vi "Send Message.vi"(8 "error in (no error)":errorcluster, 10 "Message":T1, 11 "UDP Ref":refnum<k16>) -> (0 "error out":errorcluster, 3 "connection ID out":refnum<k16>)   [LabVIEW 2019]
uses:
  Message Globals.vi
  Typedefs/Sensor Types.ctl
  Typedefs/Message Types.ctl
  Typedefs/Message.ctl
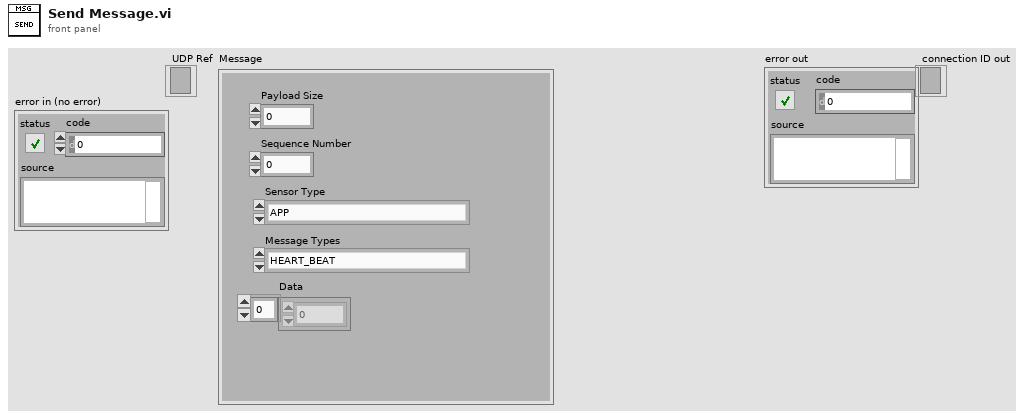
[diagram p1: front panel]
types:
  T1 = typedef "Message.ctl" = cluster{"Payload Size":u8, "Sequence Number":u8, "Sensor Type":T2, "Message Types":T3, "Data":u8[]}
  T2 = typedef "Sensor Types.ctl" = enum16{"APP", "TURBIDITY", "PH"}
  T3 = typedef "Message Types.ctl" = enum16{"HEART_BEAT", "CONNECT", "GET_CURRENT_MEASUREMENTS", "GET_LOG_FILE", "SEND_LOG_FILE_SIZE", "SEND_LOG_FILE_CHUNK", "GET_LOGGING_PERIOD", "SET_LOGGING_PERIOD", "SEND_SD_CARD_INFO", "GET_LOGS_LIST", "SEND_LOG_FILE_NAME", "SEND_LOGGING_PERIOD", "GET_RTC_TIME", "SET_RTC_TIME", "SEND_RTC_TIME", "SEND_CURRENT_MEASUREMENTS", "DELETE_LOG_FILE", "GET_SD_CARD_INFO", "GET_BATTERY_INFO", "SEND_BATTERY_INFO", "GET_LOG_FILE_SIZE", "ERROR_MSG"}
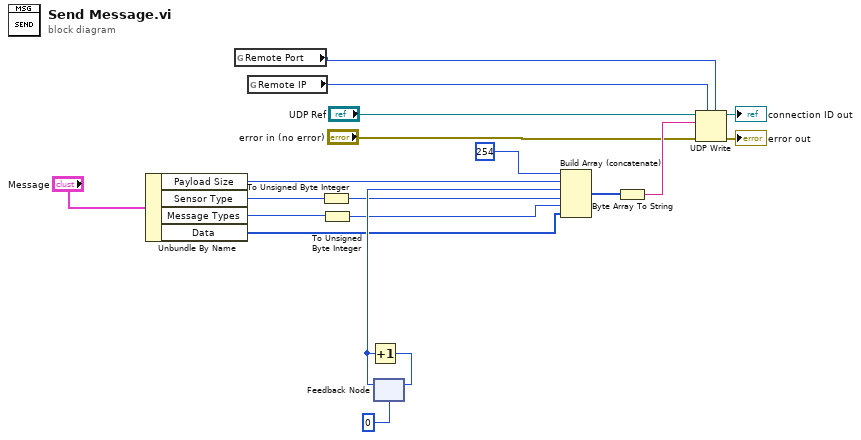
[diagram p0: block diagram]
diagram:
  n1 = Unbundle By Name("Message") -> ("Payload Size"=w9:u8, "Sensor Type"=w5:T2, "Message Types"=w3:T3, "Data"=w1:u8[])
  n2 = global read "Message Globals.vi" "Remote Port"() -> (w13:u16)
  n3 = global read "Message Globals.vi" "Remote IP"() -> (w14:u32)
  n4 = To Unsigned Byte Integer(number=w5) -> (unsigned 8bit integer=w4:u8)
  n5 = To Unsigned Byte Integer(number=w3) -> (unsigned 8bit integer=w2:u8)
  n6 = feedback #1(u8 0 ("Payload Size")) -> (w6:u8)
  n7 = Increment(x=w6) -> (x+1=w7:u8)
  n8 = feedback-in #1(w7) -> ()
  n9 = Build Array (concatenate)(u8 254 ("element"), w9, w6, w4, w2, w1) -> (w18:u8[])
  n10 = Byte Array To String(unsigned byte array=w18) -> (string=w17:string)
  n11 = UDP Write(address=w14, port or service name=w13, connection ID="UDP Ref", data in=w17, 8:"error in (no error)") -> (error out=→"error out":errorcluster, 3:→"connection ID out":refnum<k16>)  [unwired: 1 in]
